vi "TotalMDptrCount.vi"(8 "error in (no error)":errorcluster) -> (0 "error out":errorcluster, 1 "# free elements in queue":i32, 2 "# elements in queue":i32, 4 "#queues":i32)   [LabVIEW 2017, in "MDPtr.lvlib" / "MDPtrMgr.lvclass"]
uses:
  MDPtrMgr.lvclass
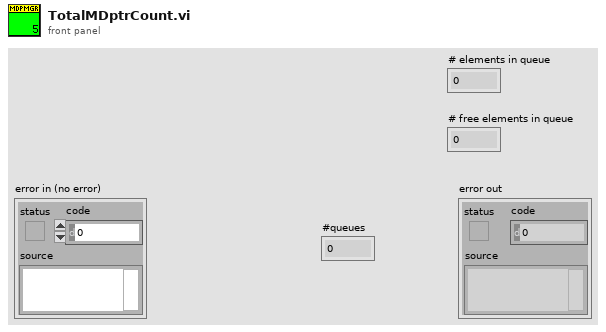
[diagram p1: front panel]
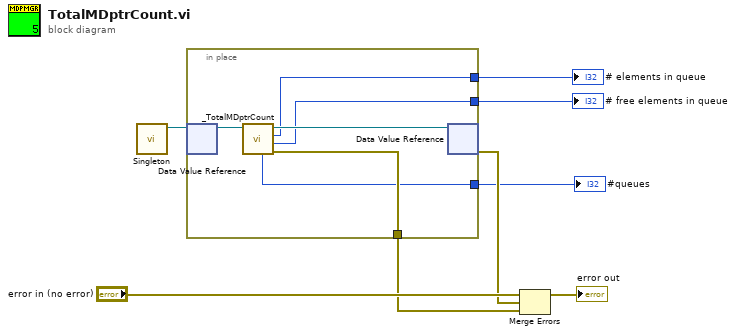
[diagram p0: block diagram]
diagram:
  n1 = call "Singleton.vi"() -> ("MDPtrMgrDVR"=w8:refnum<data-value>)  [unwired: 10 in, 1 out]
  n2 = in-place {
    in-place-border: [w12] -> w4
    in-place-border: [w11] -> w3
    in-place-border: [w10] -> w2
    in-place-border: [w9] -> w1
    n3 = in-place-dvr #1(w8) -> (w14:refnum<class "MDPtrMgr.lvclass">)  [unwired: 1 out]
    n4 = call "_TotalMDptrCount.vi"("MDPtrMgr in"=w14) -> ("error out"=w12:errorcluster, "# free elements in queue"=w10:i32, "# elements in queue"=w11:i32, "MDPtrMgr out"=w13:refnum<class "MDPtrMgr.lvclass">, "#queues"=w9:i32)  [unwired: 6 in]
    n5 = in-place-dvr #1(w13) -> (w5:errorcluster)  [unwired: 1 out]
  }
  "# elements in queue" <- w3
  "# free elements in queue" <- w2
  "#queues" <- w1
  n6 = Merge Errors("error in (no error)", w5, w4) -> (→"error out":errorcluster)
